vi "SUB-BLE Rx data (Mon)-CDC IMU.vi"(8 "data in":u8[](array[numeric]) format="%2x") -> (0 "IMU data":T1 caption="IMU Monitoring data" {"Accelerometer Z" format="%#.9f"; "Accelerometer Y" format="%#.9f"; "Accelerometer X" format="%#.9f"; "Gyroscope Z" format="%#.9f"; "Gyroscope Y" format="%#.9f"; "Gyroscope X" format="%#.9f"}, 1 "CDC data":T2 caption="CDC Monitoring data" {"Right Wing-C, C6/C0" format="%#.9f"; "Right Wing-B, C5/C0" format="%#.9f"; "Right Wing-A, C4/C0" format="%#.9f"; "Left Wing-C, C3/C0" format="%#.9f"; "Left Wing-B, C2/C0" format="%#.9f"; "Left Wing-A, C1/C0" format="%#.9f"}, 2 "Bat":u16, 3 "*Board ID":string="None...." caption="S/N")   [LabVIEW 2015]
doc: "Use this template to create an application that executes repeatedly until you click the Stop button. This template polls the state of the Stop button and does not use events. Use the Top-Level Application template (not available in the Base package) to create a single-loop application with event handling."
uses:
  Control-CDC data.ctl
  Control-IMU data.ctl
panel:
  out "원소":u8
  out "BLE Packet (buf)":u8[](array[numeric])
  out "BLE Packet (data)":u8[](array[numeric])
  # "BLE 수신 데이터를 분류: Monitoring/Setting data"
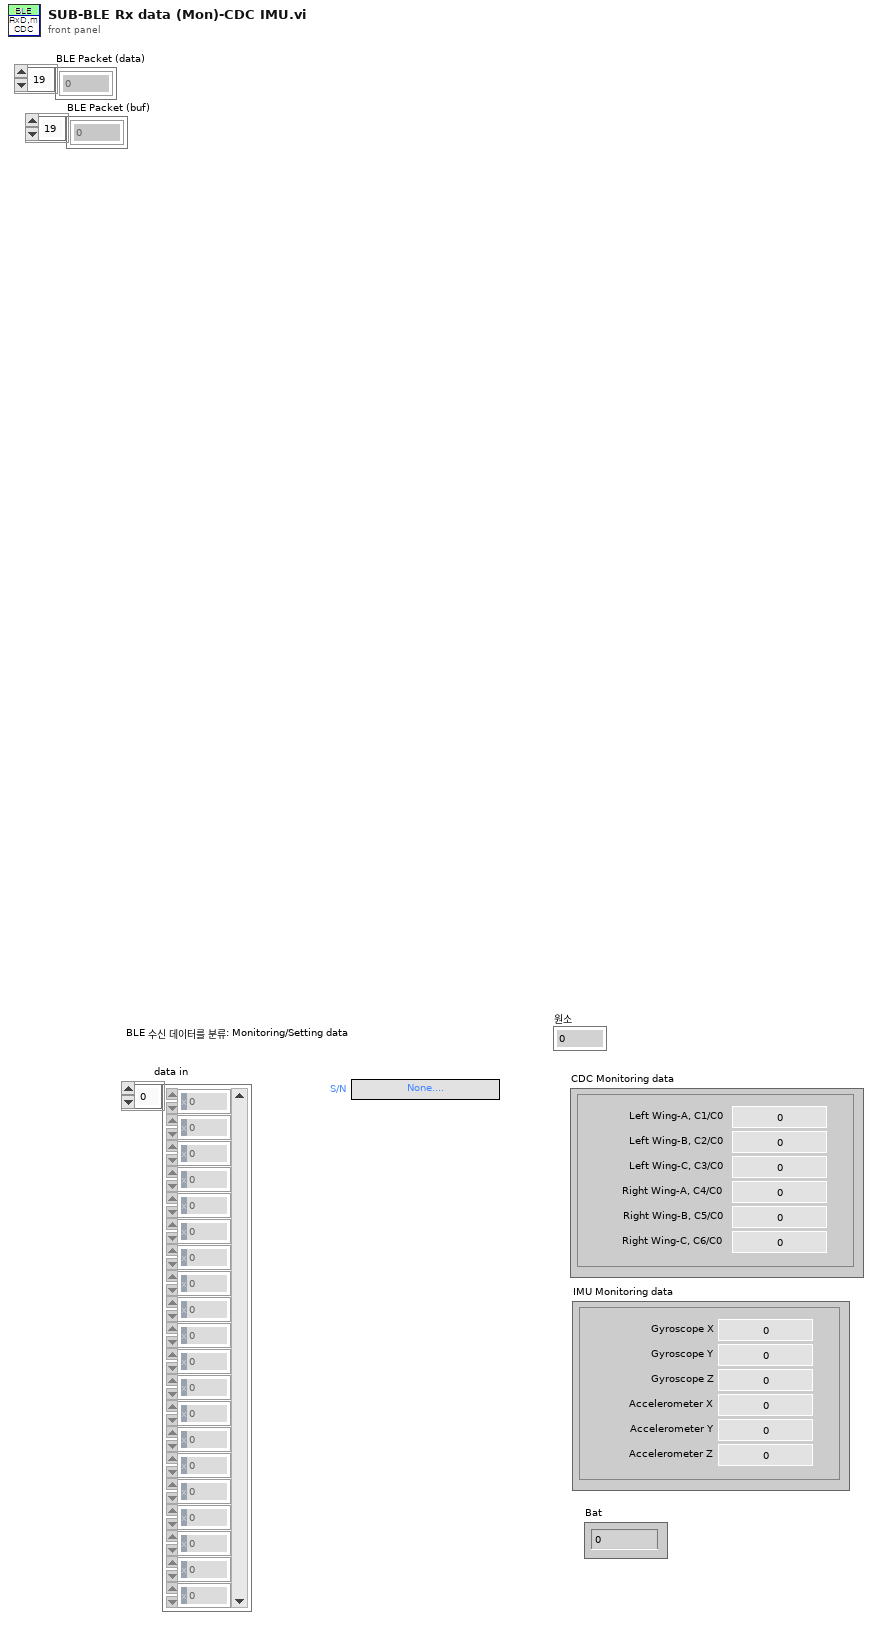
[diagram p1: front panel]
types:
  T1 = typedef "Control-IMU data.ctl" = cluster{"Gyroscope X":dbl, "Gyroscope Y":dbl, "Gyroscope Z":dbl, "Accelerometer X":dbl, "Accelerometer Y":dbl, "Accelerometer Z":dbl}
  T2 = typedef "Control-CDC data.ctl" = cluster{"Left Wing-A, C1/C0":dbl, "Left Wing-B, C2/C0":dbl, "Left Wing-C, C3/C0":dbl, "Right Wing-A, C4/C0":dbl, "Right Wing-B, C5/C0":dbl, "Right Wing-C, C6/C0":dbl}
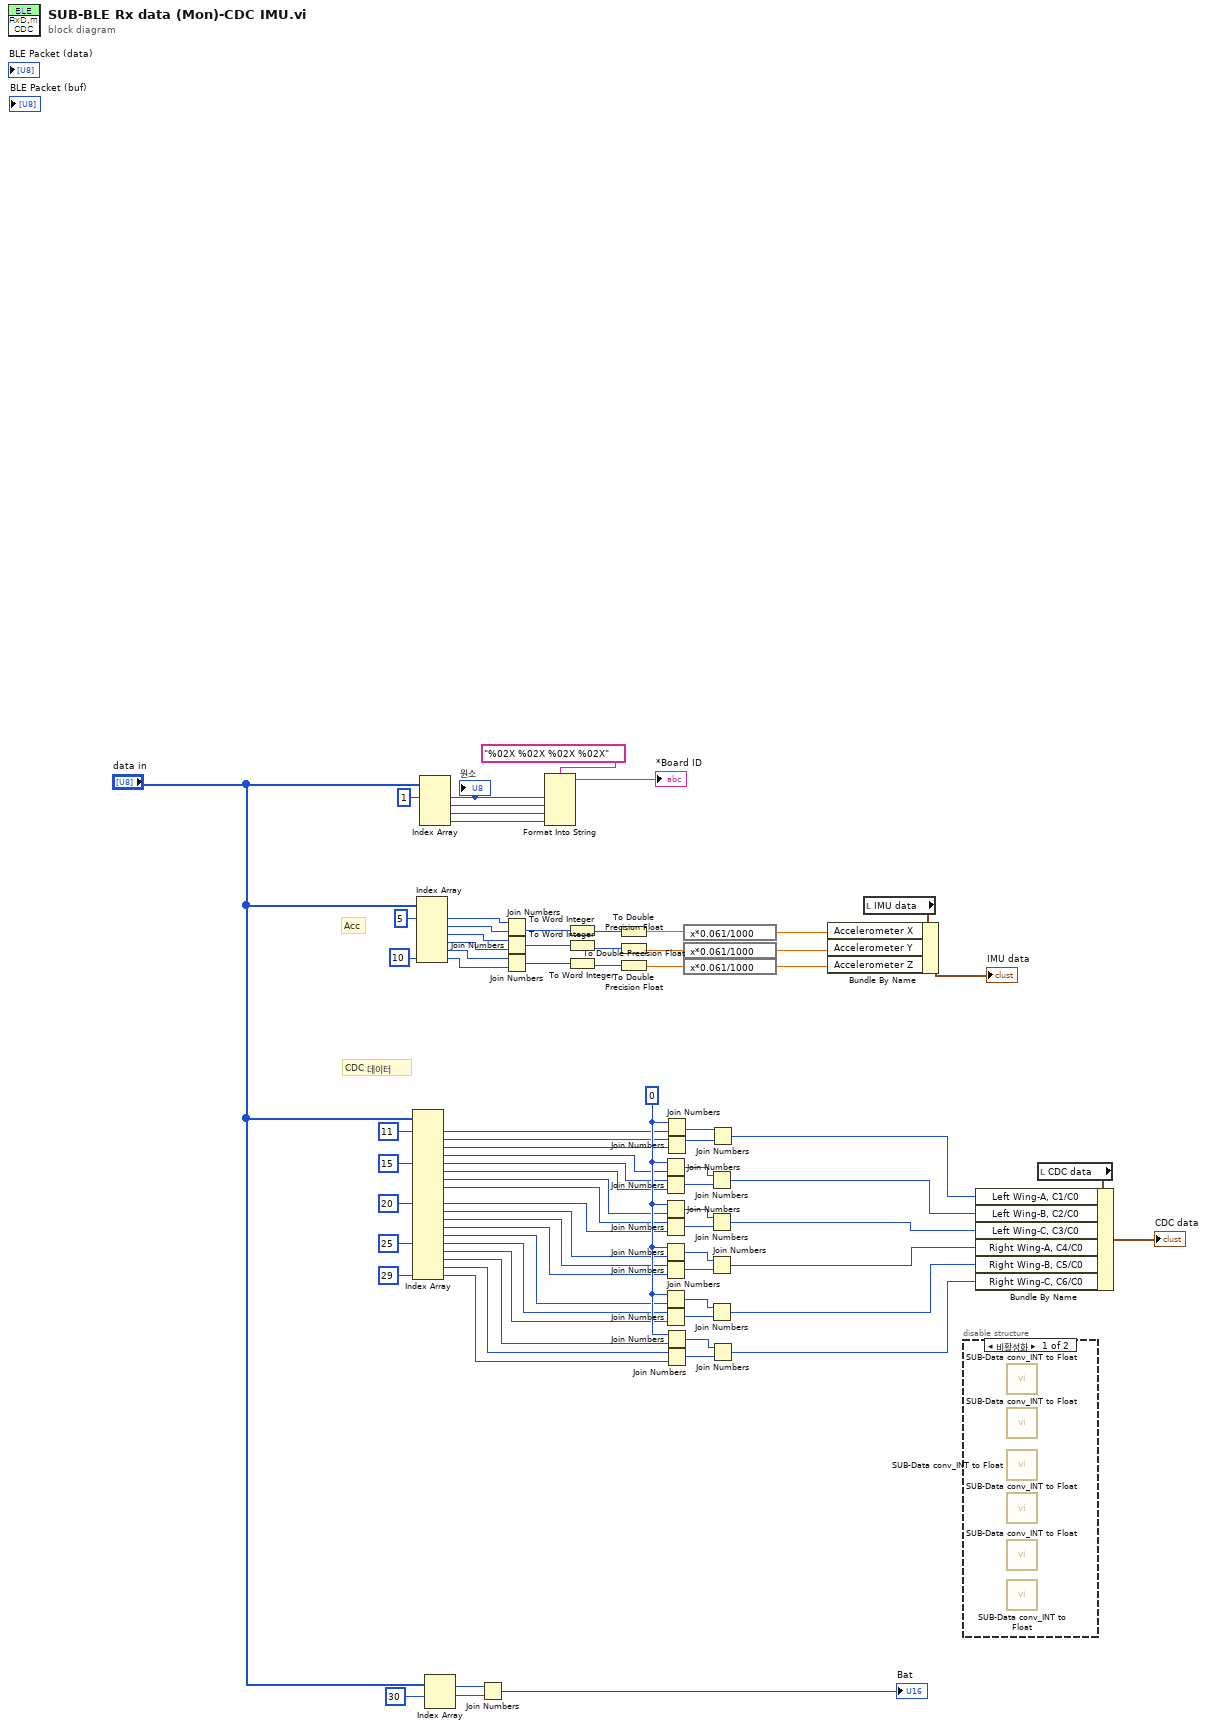
[diagram p0: block diagram]
diagram:
  w29 = u8 0 ("hi")
  # "Acc"
  # "CDC 데이터"
  n1 = Index Array(array="data in", index #1=11 ("인덱스"), index #5=15 ("인덱스"), index #10=20 ("인덱스"), index #15=25 ("인덱스"), index #19=29 ("인덱스")) -> (element #1=w28:u8, element #2=w27:u8, element #3=w26:u8, element #4=w25:u8, element #5=w24:u8, element #6=w23:u8, element #7=w22:u8, element #8=w21:u8, element #10=w16:u8, element #11=w15:u8, element #12=w14:u8, element #13=w13:u8, element #14=w12:u8, element #15=w11:u8, element #16=w10:u8, element #17=w9:u8, element #18=w8:u8, element #19=w7:u8)  [unwired: 14 in, 1 out]
  n2 = Index Array(array="data in", index #1=5 ("인덱스"), index #6=10 ("인덱스")) -> (element #1=w49:u8, element #2=w48:u8, element #3=w47:u8, element #4=w46:u8, element #5=w45:u8, element #6=w44:u8)  [unwired: 4 in]
  n3 = Index Array(array="data in", index #1=1 ("인덱스")) -> (element #1=w76:u8, element #2=w75:u8, element #3=w74:u8, element #4=w73:u8)  [unwired: 3 in]
  "원소" <- w76
  n4 = Index Array(array="data in", index #1=30 ("인덱스")) -> (element #1=w62:u8, element #2=w63:u8)  [unwired: 1 in]
  n5 = Join Numbers(hi=w62, lo=w63) -> ((hi.lo)=→"Bat":u16)
  n6 = Join Numbers(hi=w49, lo=w48) -> ((hi.lo)=w56:u16)
  n7 = Join Numbers(hi=w47, lo=w46) -> ((hi.lo)=w55:u16)
  n8 = Join Numbers(hi=w45, lo=w44) -> ((hi.lo)=w54:u16)
  n9 = Format Into String(format string="%02X %02X %02X %02X" ("구분 문자(탭)"), w76, w75, w74, w73) -> (resulting string=→"*Board ID":string)  [unwired: 2 in, 1 out]
  n10 = To Word Integer(number=w56) -> (16bit integer=w59:i16)
  n11 = To Word Integer(number=w55) -> (16bit integer=w58:i16)
  n12 = To Word Integer(number=w54) -> (16bit integer=w57:i16)
  n13 = To Double Precision Float(number=w59) -> (double precision float=w67:dbl)
  n14 = To Double Precision Float(number=w58) -> (double precision float=w66:dbl)
  n15 = To Double Precision Float(number=w57) -> (double precision float=w65:dbl)
  n16 = Join Numbers(hi=w29, lo=w25) -> ((hi.lo)=w39:u16)
  n17 = Join Numbers(hi=w24, lo=w23) -> ((hi.lo)=w38:u16)
  n18 = Join Numbers(hi=w29, lo=w22) -> ((hi.lo)=w36:u16)
  n19 = Join Numbers(hi=w21, lo=w16) -> ((hi.lo)=w37:u16)
  n20 = Join Numbers(hi=w29, lo=w15) -> ((hi.lo)=w35:u16)
  n21 = Join Numbers(hi=w14, lo=w13) -> ((hi.lo)=w34:u16)
  n22 = Join Numbers(hi=w29, lo=w12) -> ((hi.lo)=w32:u16)
  n23 = Join Numbers(hi=w11, lo=w10) -> ((hi.lo)=w33:u16)
  n24 = Join Numbers(hi=w29, lo=w28) -> ((hi.lo)=w40:u16)
  n25 = Join Numbers(hi=w27, lo=w26) -> ((hi.lo)=w41:u16)
  n26 = Join Numbers(hi=w29, lo=w9) -> ((hi.lo)=w31:u16)
  n27 = Join Numbers(hi=w8, lo=w7) -> ((hi.lo)=w30:u16)
  n28 = expression code="x*0.061/1000"(w67) -> (w52:dbl)
  n29 = expression code="x*0.061/1000"(w66) -> (w51:dbl)
  n30 = expression code="x*0.061/1000"(w65) -> (w50:dbl)
  n31 = Join Numbers(hi=w39, lo=w38) -> ((hi.lo)=w5:u32)
  n32 = Join Numbers(hi=w36, lo=w37) -> ((hi.lo)=w4:u32)
  n33 = Join Numbers(hi=w35, lo=w34) -> ((hi.lo)=w3:u32)
  n34 = Join Numbers(hi=w32, lo=w33) -> ((hi.lo)=w2:u32)
  n35 = Join Numbers(hi=w40, lo=w41) -> ((hi.lo)=w6:u32)
  n36 = Join Numbers(hi=w31, lo=w30) -> ((hi.lo)=w1:u32)
  n37 = local read "IMU data"() -> (w68:T1)
  n38 = Bundle By Name(cluster=w68, "Accelerometer X"=w52, "Accelerometer Y"=w51, "Accelerometer Z"=w50) -> (→"IMU data":T1)
  n39 = disable-structure shown="비활성화" {
    frame Disabled {
      n40 = call "SUB-Data conv_INT to Float.vi"() -> ()  [unwired: 3 in, 1 out]
      n41 = call "SUB-Data conv_INT to Float.vi"() -> ()  [unwired: 3 in, 1 out]
      n42 = call "SUB-Data conv_INT to Float.vi"() -> ()  [unwired: 3 in, 1 out]
      n43 = call "SUB-Data conv_INT to Float.vi"() -> ()  [unwired: 3 in, 1 out]
      n44 = call "SUB-Data conv_INT to Float.vi"() -> ()  [unwired: 3 in, 1 out]
      n45 = call "SUB-Data conv_INT to Float.vi"() -> ()  [unwired: 3 in, 1 out]
    }
    frame Enabled {
    }
  }
  n46 = local read "CDC data"() -> (w71:T2)
  n47 = Bundle By Name(cluster=w71, "Left Wing-A, C1/C0"=w6, "Left Wing-B, C2/C0"=w5, "Left Wing-C, C3/C0"=w4, "Right Wing-A, C4/C0"=w3, "Right Wing-B, C5/C0"=w2, "Right Wing-C, C6/C0"=w1) -> (→"CDC data":T2)
